vi "RankNodes.vi"(9 "VI_AST in":refnum<class "VI_Hierarchy.lvclass">) -> (3 "VI_AST out":refnum<class "VI_Hierarchy.lvclass">, 4 "Rank":cluster{"nodes":string[]}[](array[cluster]))   [LabVIEW 2014, in "VI_Hierarchy.lvclass"]
uses:
  VI_Hierarchy.lvclass
  VI_Hierarchy.lvclass/VI_Hierarchy.ctl
  DAG/DAG/DAG.lvclass
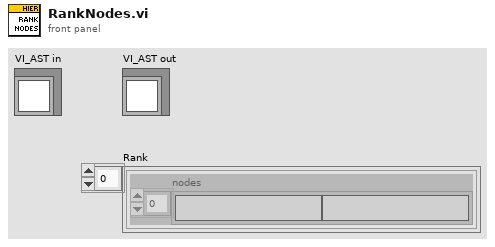
[diagram p1: front panel]
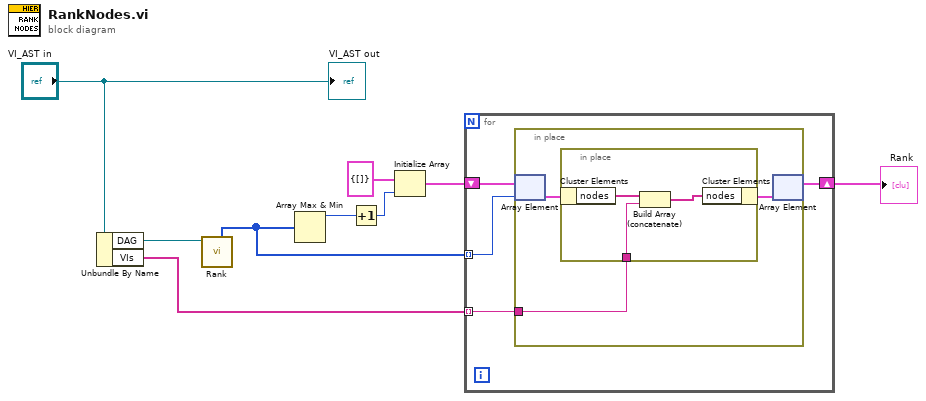
[diagram p0: block diagram]
diagram:
  n1 = Unbundle By Name("VI_AST in") -> ("DAG"=w8:refnum<class "DAG.lvclass">, "VIs"=w2:string[])
  n2 = call "Rank.vi"("DAG in"=w8) -> ("rank"=w3:i32[])  [unwired: 8 in]
  n3 = Array Max & Min(array=w3) -> (max value=w6:i32)  [unwired: 3 out]
  n4 = Increment(x=w6) -> (x+1=w5:i32)
  n5 = Initialize Array(cluster{"nodes":string[]} {"nodes"=[]}, w5) -> (w4:cluster{"nodes":string[]}[])
  n6 = for {
    shift-right: [w11] -> w1
    shift-left: w4 -> [w13]
    tunnel: w2 -> [w10] mode=indexing
    tunnel: w3 -> [w12] mode=indexing
    n7 = in-place {
      in-place-border: w10 -> [w14]
      n8 = in-place-array #1(w13, w12) -> (w16:cluster{"nodes":string[]})
      n9 = in-place {
        in-place-border: w14 -> [w17]
        n10 = in-place-cluster #2(w16) -> ("nodes"=w19:string[])
        n11 = Build Array (concatenate)(w19, w17) -> (w18:string[])
        n12 = in-place-cluster #2("nodes"=w18) -> (w15:cluster{"nodes":string[]})
      }
      n13 = in-place-array #1(w15) -> (w11:cluster{"nodes":string[]}[])  [unwired: 1 out]
    }
  }
  "Rank" <- w1
  "VI_AST out" <- "VI_AST in"
